vi "Configure Serial Bus (Flexray - Trigger - Event Autoset).vi"(0 "VISA resource name":refnum<visa-resource-name>, 5 "Serial Bus Name (1: Serial Bus 1)":i32(ring)=1 items=["Serial Bus 1"=1, "Serial Bus 2"=2], 11 "error in (no error)":errorcluster) -> (4 "VISA resource name out":refnum<visa-resource-name>, 15 "error out":errorcluster)   [LabVIEW 2023, in "Keysight-DSQx3014T.lvlib"]
doc: "Configures oscilloscope settings (as shown on the display) for the selected event trigger automatically."
uses:
  Keysight-DSQx3014T.lvlib
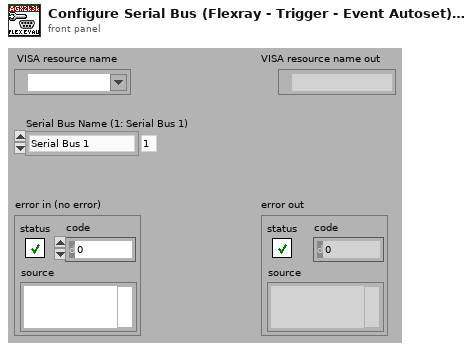
[diagram p1: front panel]
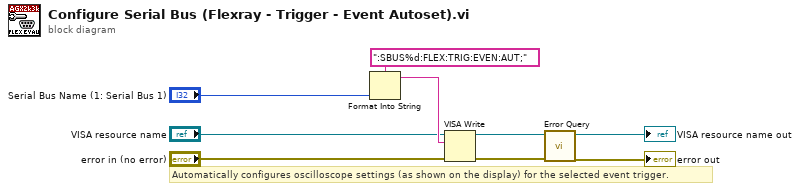
[diagram p0: block diagram]
diagram:
  # "Automatically configures oscilloscope settings (as shown on the display) for the selected event trigger."
  n1 = Format Into String(format string=":SBUS%d:FLEX:TRIG:EVEN:AUT;", "Serial Bus Name (1: Serial Bus 1)") -> (resulting string=w7:string)  [unwired: 2 in, 1 out]
  n2 = VISA Write(VISA resource name="VISA resource name", write buffer=w7, error in (no error)="error in (no error)") -> (VISA resource name out=w4:refnum<visa-resource-name>, error out=w3:errorcluster)  [unwired: 1 out]
  n3 = call "Error Query.vi"("error in (no error)"=w3, "VISA resource name"=w4) -> ("error out"=→"error out":errorcluster, "VISA resource name out"=→"VISA resource name out":refnum<visa-resource-name>)  [unwired: 8 out]
